vi "CI_Facade.vi"(0 "Data In":T4, 2 "Display State In":T2={"StandardColor"=0, "WarningColor"=15671808, "CriticalColor"=15671808, "Standard<>Warning Range"=0, "Warning<>Critical Range"=0}, 3 "Container State":T3) -> (6 "Data Out":T4, 7 "Display State Out":T2={"StandardColor"=0, "WarningColor"=15671808, "CriticalColor"=15671808, "Standard<>Warning Range"=0, "Warning<>Critical Range"=0}, 8 "Action":T1)   [LabVIEW 2010, in "CapacityIndicator.xctl"]
doc: "Use capacity indicator to provide information about the level or amount of something that has well defined minimum and maximum values. For example, you might use a capacity indicator to showthe current level of storage-space usage on a server or the charge left in a battery.\n\nCopyright 2007 SAPHIR (Olivier JOURDAN) All Rights Reserved"
uses:
  CapacityIndicator.xctl
  CI_Data.ctl
  <vilib>/_xctls/Container State.ctl
  CI_State.ctl
  <vilib>/_xctls/Action.ctl
  <vilib>/_xctls/XControlSupport.lvlib
panel:
  in  "Capacity":u8(slide) scale=0.0..100.0
  # "1. Drop the controls that make up the appearance\nof the XControl here.\n\n2. Resize the window to fit the controls\n\n3. If the XControl is of fixed size,  make the \n window not resizable from VI Properties->Window Appearance.\n\n4. If you want the controls to automatically size when the XControl sizes, check  \"Scale all objects on front panel when window resizes\" in File->VI Properties->Window Size page.\n\n5. Show the block diagram and handle events for the controls on this panel."
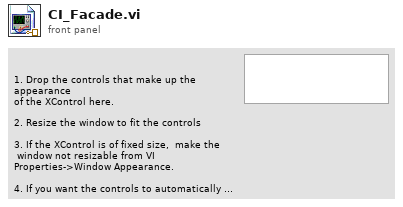
[diagram p1: front panel]
types:
  T1 = typedef "XControlSupport.lvlib/Action.ctl" = cluster{"Data Changed?":bool, "State Changed?":bool, "Action Name":string}
  T2 = typedef "CapacityIndicator.xctl/CI_State.ctl" = cluster{"StandardColor":u32, "WarningColor":u32, "CriticalColor":u32, "Standard<>Warning Range":u8, "Warning<>Critical Range":u8}
  T3 = typedef "XControlSupport.lvlib/Container State.ctl" = cluster{"Indicator?":bool, "Run Mode?":bool, " Refnum":refnum<vi>}
  T4 = typedef "CapacityIndicator.xctl/CI_Data.ctl" = u8
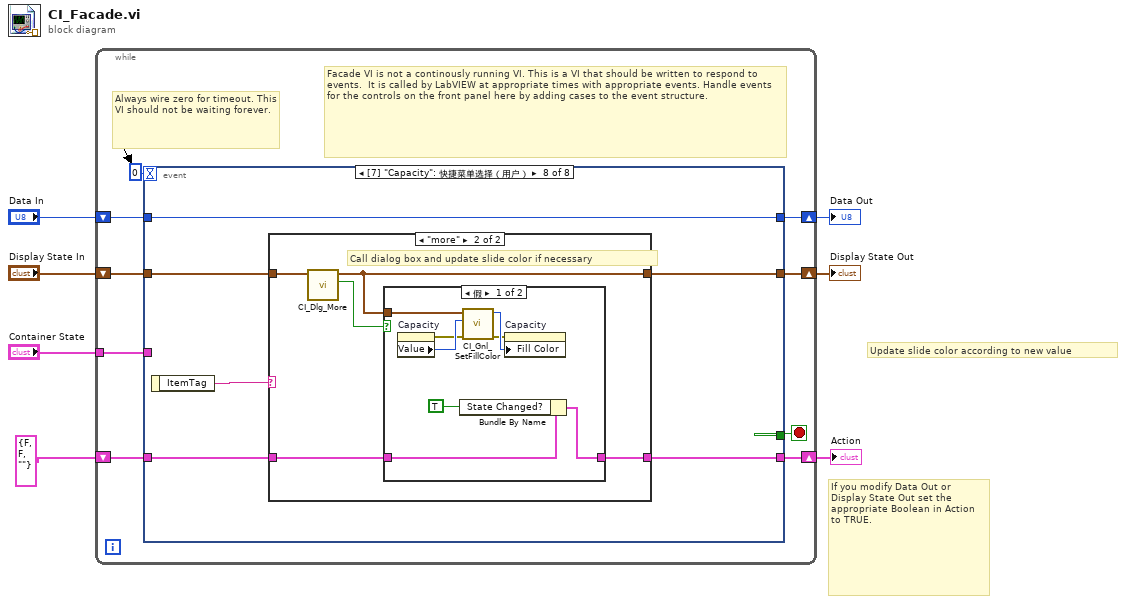
[diagram p0: block diagram]
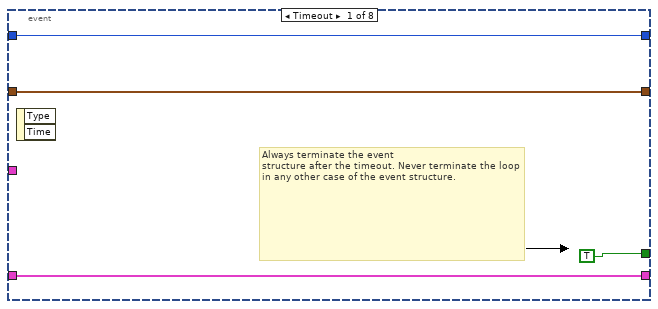
[diagram p2: hidden frame]
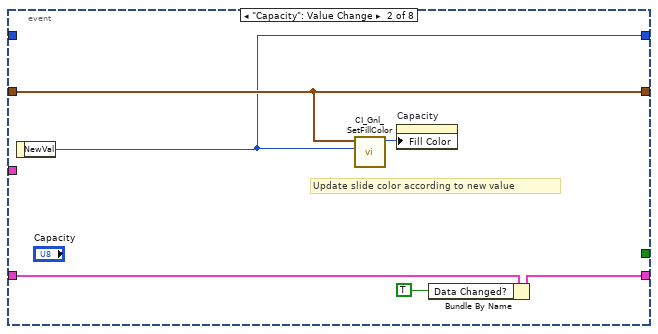
[diagram p3: hidden frame]
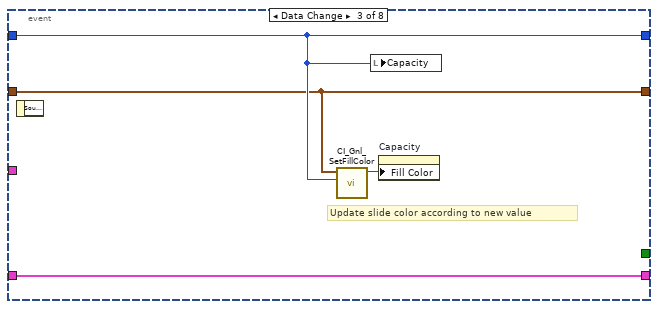
[diagram p4: hidden frame]
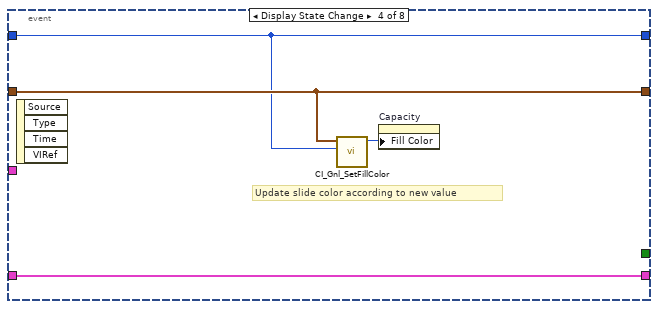
[diagram p5: hidden frame]
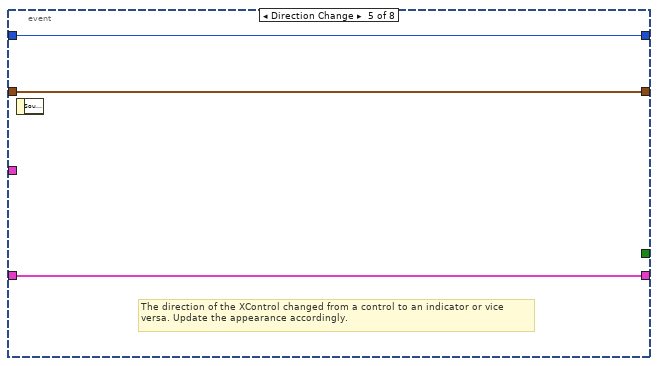
[diagram p6: hidden frame]
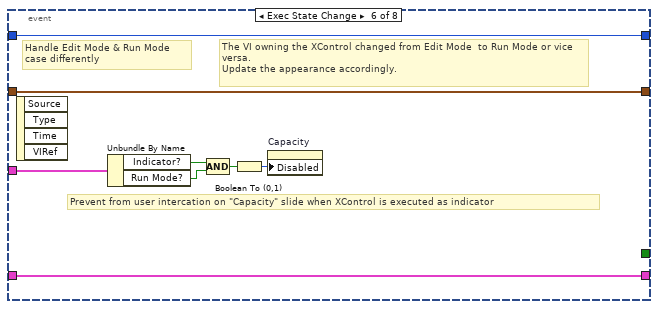
[diagram p7: hidden frame]
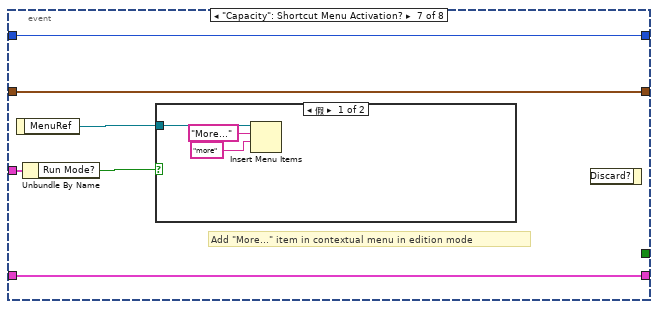
[diagram p8: hidden frame]
diagram:
  # "Update slide color according to new value"
  # "If you modify Data Out or\nDisplay State Out set the\nappropriate Boolean in Action\nto TRUE."
  n1 = while {
    shift-right: [w15] -> w4
    shift-left: "Display State In" -> [w16]
    tunnel: "Container State" -> [w12]
    shift-right: [w10] -> w7
    shift-left: "Data In" -> [w11]
    shift-right: [w8] -> w2
    shift-left: T1 {"Data Changed?"=FALSE, "State Changed?"=FALSE, "Action Name"=""} ("Action") -> [w9]
    stop <- w14 stop-if-true
    # "Facade VI is not a continously running VI. This is a VI that should be written to respond to events.  It is called by LabVIEW at appropriate times with appropriate events. Handle events for the controls on the front panel here by adding cases to the event structure."
    # "Always wire zero for timeout. This\nVI should not be waiting forever."
    n2 = event shown="[7] \"Capacity\": 快捷菜单选择（用户）" {
      selector: _ -> [_ _ _ _ _ _ _ _]
      dyn-events: _ -> [_ _ _ _ _ _ _ _]
      timeout: 0 -> [_ _ _ _ _ _ _ _]
      tunnel: w16 -> [w18 w22 w27 w32 w37 w45 w47 w59]
      tunnel: [w18 w22 w27 w32 w37 w45 w47 w57] -> w15
      tunnel: [TRUE _ _ _ _ _ _ _] -> w14
      tunnel: w12 -> [_ _ _ _ _ w38 w51 _]
      tunnel: w11 -> [w17 _ w28 w31 w36 w44 w48 w60]
      tunnel: [w17 w21 w28 w31 w36 w44 w48 w60] -> w10
      tunnel: [w19 w25 w30 w34 w35 w43 w46 w56] -> w8
      tunnel: w9 -> [w19 w26 w30 w34 w35 w43 w46 w55]
      event Timeout {
        # "Always terminate the event\nstructure after the timeout. Never terminate the loop in any other case of the event structure."
        n3 = event-data() -> ()  [unwired: 1 in, 2 out]
      }
      event "Capacity": Value Change {
        # "Update slide color according to new value"
        n4 = event-data() -> ("NewVal"=w21:u8)  [unwired: 1 in]
        n5 = call "CI_Gnl_SetFillColor.vi"("Value"=w21, "Display State In"=w22) -> ("FillColor"=w23:u32)  [unwired: 8 in, 1 out]
        n6 = property on="Capacity" class="Slide (严格)"("Fill Color"=w23) -> ()  [unwired: 2 in, 2 out]
        n7 = Bundle By Name(cluster=w26, "Data Changed?"=TRUE) -> (w25:T1)
      }
      event Data Change {
        # "Update slide color according to new value"
        n8 = event-data() -> ()  [unwired: 1 in, 1 out]
        n9 = call "CI_Gnl_SetFillColor.vi"("Value"=w28, "Display State In"=w27) -> ("FillColor"=w29:u32)  [unwired: 8 in, 1 out]
        n10 = local write "Capacity"(w28) -> ()
        n11 = property on="Capacity" class="Slide (严格)"("Fill Color"=w29) -> ()  [unwired: 2 in, 2 out]
      }
      event Display State Change {
        # "Update slide color according to new value"
        n12 = event-data() -> ()  [unwired: 1 in, 4 out]
        n13 = call "CI_Gnl_SetFillColor.vi"("Value"=w31, "Display State In"=w32) -> ("FillColor"=w33:u32)  [unwired: 8 in, 1 out]
        n14 = property on="Capacity" class="Slide (严格)"("Fill Color"=w33) -> ()  [unwired: 2 in, 2 out]
      }
      event Direction Change {
        # "The direction of the XControl changed from a control to an indicator or vice versa. Update the appearance accordingly."
        n15 = event-data() -> ()  [unwired: 1 in, 1 out]
      }
      event Exec State Change {
        # "Prevent from user intercation on \"Capacity\" slide when XControl is executed as indicator"
        # "The VI owning the XControl changed from Edit Mode  to Run Mode or vice versa.\nUpdate the appearance accordingly."
        # "Handle Edit Mode & Run Mode\ncase differently"
        n16 = event-data() -> ()  [unwired: 1 in, 4 out]
        n17 = Unbundle By Name(w38) -> ("Indicator?"=w41:bool, "Run Mode?"=w39:bool)
        n18 = Compound Arithmetic op=AND(w41, w39) -> (w40:bool)
        n19 = Boolean To (0,1)(Boolean=w40) -> (0, 1=w42:i16)
        n20 = property on="Capacity" class="Slide (严格)"("Disabled"=w42) -> ()  [unwired: 2 in, 2 out]
      }
      event "Capacity": Shortcut Menu Activation? {
        # "Add \"More...\" item in contextual menu in edition mode"
        n21 = event-data() -> ("MenuRef"=w49:refnum<k9>)  [unwired: 1 in]
        n22 = Unbundle By Name(w51) -> ("Run Mode?"=w50:bool)
        n23 = case shown="假" w50 {
          tunnel: w49 -> [w54 _]
          frame False {
            n24 = Insert Menu Items(7:"more", 8:"More...", 9:w54) -> ()  [unwired: 3 in, 3 out]
          }
          frame True {
          }
        }
        n25 = event-data() -> ()  [unwired: 2 in, 1 out]
      }
      event "Capacity": Shortcut Menu Selection (User) {
        n26 = event-data() -> ("ItemTag"=w58:string)  [unwired: 1 in]
        n27 = case shown="\"more\"" w58 {
          tunnel: w59 -> [w62 w67]
          tunnel: [w62 w66] -> w57
          tunnel: [w61 w63] -> w56
          tunnel: w55 -> [w61 w64]
          frame Default {
          }
          frame "more" {
            # "Call dialog box and update slide color if necessary"
            n28 = call "CI_Dlg_More.vi"("Display State In"=w67) -> ("Cancel?"=w65:bool, "Display State Out"=w66:T2)  [unwired: 8 in, 1 out]
            n29 = case shown="假" w65 {
              tunnel: w66 -> [w71 _]
              tunnel: w64 -> [w69 w76]
              tunnel: [w68 w76] -> w63
              frame False {
                n30 = property on="Capacity" class="Slide (严格)"() -> (error out=w73:errorcluster, "Value"=w74:u8)  [unwired: 2 in, 1 out]
                n31 = Bundle By Name(cluster=w69, "State Changed?"=TRUE) -> (w68:T1)
                n32 = call "CI_Gnl_SetFillColor.vi"("error in"=w73, "Value"=w74, "Display State In"=w71) -> ("error out"=w72:errorcluster, "FillColor"=w75:u32)  [unwired: 7 in]
                n33 = property on="Capacity" class="Slide (严格)"(error in=w72, "Fill Color"=w75) -> ()  [unwired: 1 in, 2 out]
              }
              frame True {
                # "Canceled"
              }
            }
          }
        }
      }
    }
  }
  "Display State Out" <- w4
  "Data Out" <- w7
  "Action" <- w2
